vi "Ex-2 RT.vi"() -> ()   [LabVIEW 2014]
uses:
  <vilib>/NI/cRIO Wfm/ChannelConfig.ctl
  <vilib>/FPGAPlugInAG/sbRIO-9651/niLvFpga_Open_sbRIO-9651.vi
  <vilib>/rvi/interface/common/dynamic/niFpgaDynamicAddResources.vi
  <vilib>/FPGAPlugInAG/Dynamic/niLvFpga_Reset_Dynamic.vi
  <vilib>/FPGAPlugInAG/Dynamic/niLvFpga_Run_Dynamic.vi
  <vilib>/Utility/error.llb/Error Cluster From Error Code.vi
  <vilib>/rvi/errors/niLvFpgaAdjustHostInterfaceError.vi
  <vilib>/NI/cRIO Wfm/AcqRead(Wfm).vi
  <vilib>/FPGAPlugInAG/Dynamic/niLvFpga_Close_Dynamic.vi
  <vilib>/rvi/interface/nirviOpenFPGA/nirviOpenFPGA.xnode
  FPGA Bitfiles/SOMHands-ON_FPGATarget_Ex-2FPGASoln_+o7aZEmXAhs.lvbitx
  <vilib>/rvi/interface/nirviMethod/nirviMethod.xnode
  <vilib>/rvi/interface/nirviReadWriteControl/nirviReadWriteControl.xnode
  <vilib>/rvi/interface/nirviCloseFPGA/nirviCloseFPGA.xnode
  <vilib>/NI/cRIO Wfm/cRIO Wfm.lvlib
  NiFpgaLv.dll
  <vilib>/rvi/interface/Simulation/niFpgaSimulationCallBeginRW.vi
panel:
  in  "SPI PHY Settings":T1={"Divide Value"=10, "Transfer Length (bits)"=16, "CS Asserted Polarity"=FALSE, "Clock Polarity (CPOL)"=FALSE, "Clock Phase (CPHA)"=FALSE, "Lengthen MISO Setup"=FALSE, "Direction Change Bit"=0, "MOSI Starts as Output"=FALSE, "Tristatable MOSI"=FALSE}
  out "Acquired Data":waveform(sgl)[](graph)
  in  "scan rate [S/s]":u32=25000
  in  "quit":bool
  in  "number of samples":i32=2000 min=128
  in  "Samples per Channel":i32=1000
  # "Channel Settings"
  # "VI Controls"
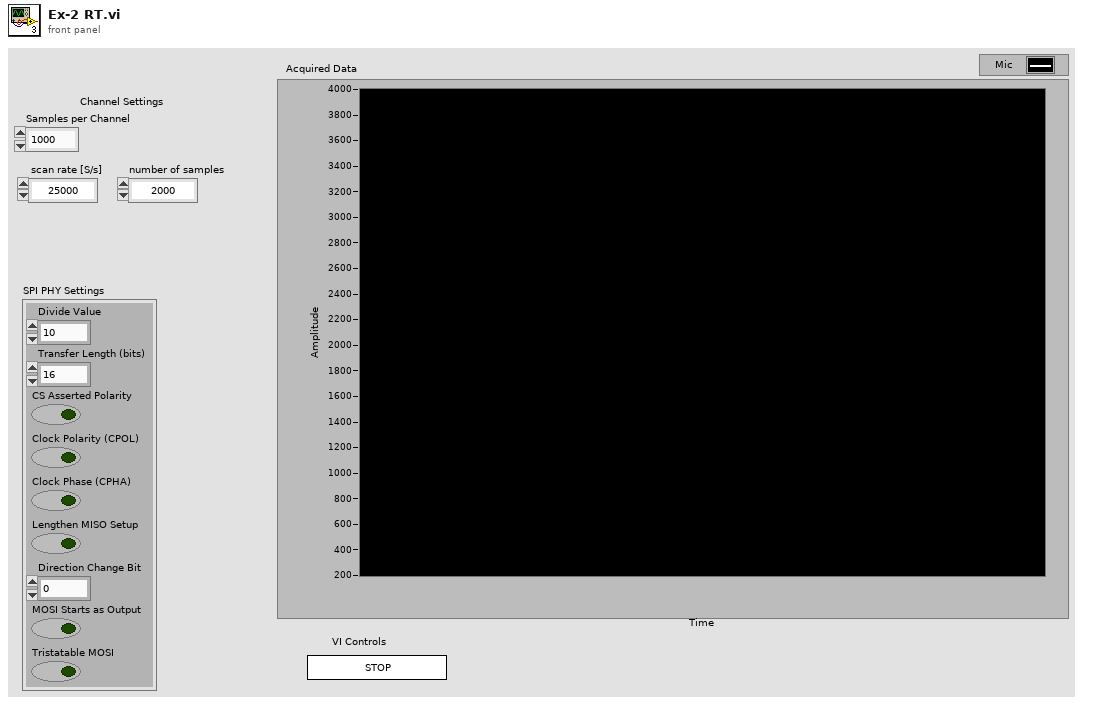
[diagram p1: front panel]
types:
  T1 = cluster{"Divide Value":u8, "Transfer Length (bits)":u8, "CS Asserted Polarity":bool, "Clock Polarity (CPOL)":bool, "Clock Phase (CPHA)":bool, "Lengthen MISO Setup":bool, "Direction Change Bit":u8, "MOSI Starts as Output":bool, "Tristatable MOSI":bool}
  T2 = typedef "cRIO Wfm.lvlib/ChannelConfig.ctl" = cluster{"Channel Name":string, "Sensitivity mV_EU":dbl, "EU":string, "dB Ref EU":dbl}[]
  T3 = typedef "cRIO Wfm.lvlib/SamplingInfo.ctl" = cluster{"Number of Channels":i32, "Actual Samp Rate":dbl, "Chan Name Array":string[], "EU Chan Array":string[], "dB Ref Chan Array":dbl[]}
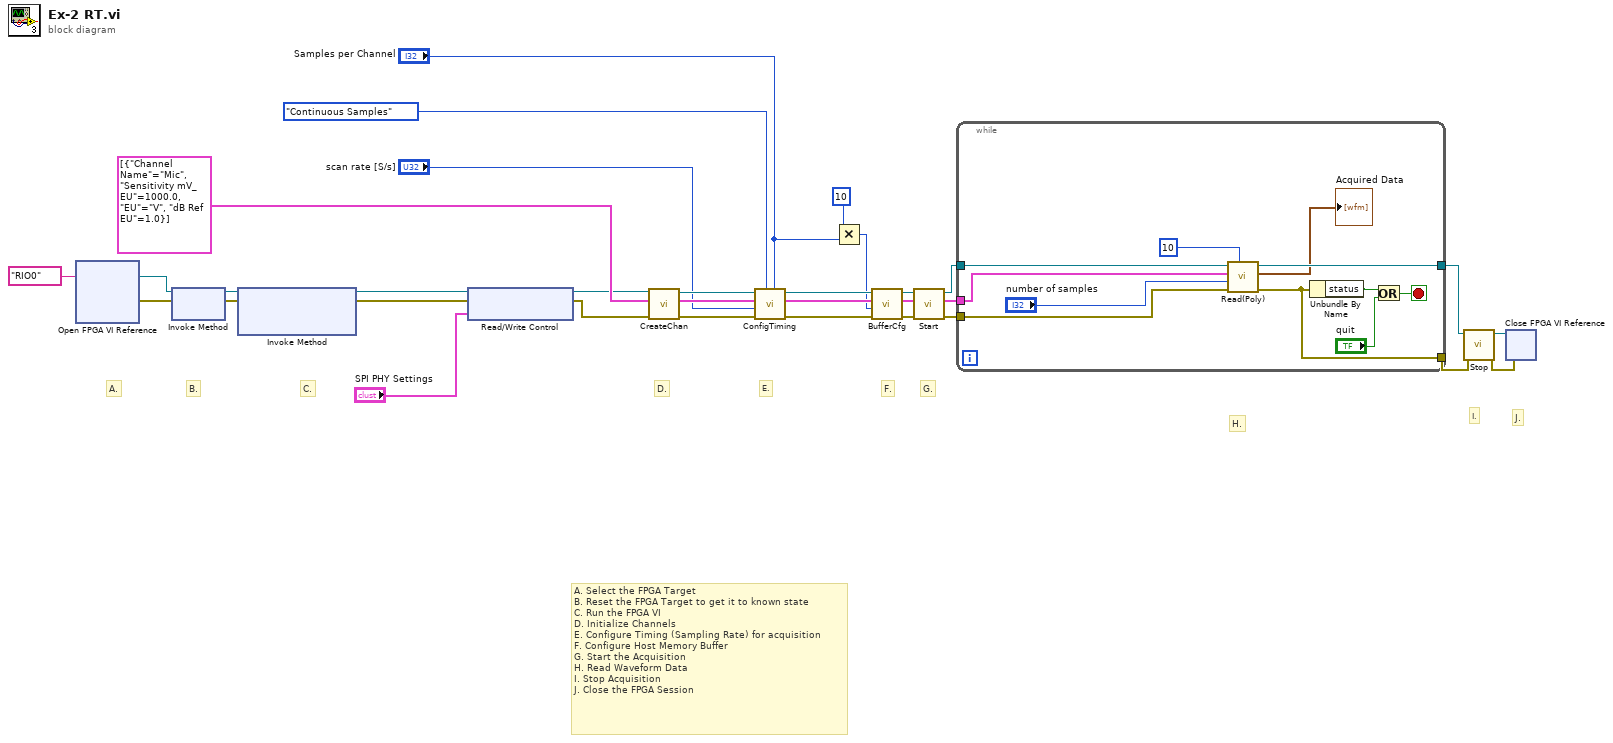
[diagram p0: block diagram]
diagram:
  # "A. Select the FPGA Target\nB. Reset the FPGA Target to get it to known state\nC. Run the FPGA VI\nD. Initialize Channels\nE. Configure Timing (Sampling Rate) for acquisition\nF. Configure Host Memory Buffer\nG. Start the Acquisition\nH. Read Waveform Data\nI. Stop Acquisition\nJ. Close the FPGA Session"
  # "J."
  # "I."
  # "H."
  # "G."
  # "F."
  # "E."
  # "D."
  # "C."
  # "B."
  # "A."
  n1 = xnode "Open FPGA VI Reference"("resource name"=tag "RIO0") -> ("FPGA VI Reference Out"=w18:refnum<k20>, "error out"=w19:errorcluster)  [unwired: 1 in]
  n2 = xnode "Invoke Method"("FPGA VI Reference In"=w18, "error in"=w19) -> ("FPGA VI Reference Out"=w17:refnum<k20>, "error out"=w16:errorcluster)
  n3 = xnode "Invoke Method"("FPGA VI Reference In"=w17, "error in"=w16) -> ("FPGA VI Reference Out"=w5:refnum<k20>, "error out"=w3:errorcluster)  [unwired: 1 in]
  n4 = xnode "Read/Write Control"("FPGA VI Reference In"=w5, "error in"=w3, "SPI PHY Settings"="SPI PHY Settings") -> ("FPGA VI Reference Out"=w4:refnum<k20>, "error out"=w2:errorcluster)
  n5 = call <vilib>:"CreateChan.vi"("error in"=w2, "Channel Info"=T2 [{"Channel Name"="Mic", "Sensitivity mV_EU"=1000.0, "EU"="V", "dB Ref EU"=1.0}], "Dynamic FPGA Ref"=w4) -> ("error out"=w22:errorcluster, "Sampling Info"=w26:T3, "Dynamic FPGA Ref Out"=w32:refnum<k20>)  [unwired: 6 in]
  n6 = call <vilib>:"ConfigTiming.vi"("Samples per Channel"="Samples per Channel", "Sample Mode"=enum16{"Finite Samples", "Continuous Samples"}."Continuous Samples", "error in"=w22, "Sample Rate"="scan rate [S/s]", "Sampling Info In"=w26, "Dynamic FPGA Ref"=w32) -> ("error out"=w21:errorcluster, "Sampling Info Out"=w27:T3, "Dynamic FPGA Ref Out"=w31:refnum<k20>)  [unwired: 2 in, 1 out]
  n7 = Multiply(x=10, y="Samples per Channel") -> (x*y=w23:i32)
  n8 = call <vilib>:"BufferCfg.vi"("error in"=w21, "Buffer Size [Samps per Chan]"=w23, "Sampling Info In"=w27, "Dynamic FPGA Ref"=w31) -> ("error out"=w20:errorcluster, "Sampling Info Out"=w25:T3, "Dynamic FPGA Ref Out"=w30:refnum<k20>)  [unwired: 4 in, 1 out]
  n9 = call <vilib>:"Start.vi"("error in"=w20, "Sampling Info In"=w25, "Dynamic FPGA Ref"=w30) -> ("error out"=w8:errorcluster, "Sampling Info Out"=w7:T3, "Dynamic FPGA Ref Out"=w9:refnum<k20>)  [unwired: 6 in]
  n10 = while {
    tunnel: [w35] -> w11
    tunnel: [w40] -> w12
    tunnel: w9 -> [w33]
    tunnel: w8 -> [w38]
    tunnel: w7 -> [w36]
    stop <- w42 stop-if-true
    n11 = call-poly <vilib>:"Read(Poly).vi"("Poll Time (ms)"=u32 10, "error in"=w38, "Samps Read per Chan"="number of samples", "Sampling Info"=w36, "Dynamic FPGA Ref"=w33) -> ("error out"=w35:errorcluster, "Wfm Data"=→"Acquired Data":waveform(sgl)[], "Dynamic FPGA Ref Out"=w40:refnum<k20>)  [unwired: 3 in, 1 out]
    n12 = Unbundle By Name(w35) -> ("status"=w41:bool)
    n13 = Or(x=w41, y="quit") -> (x .or. y?=w42:bool)
  }
  n14 = call <vilib>:"Stop.vi"("error in"=w11, "Dynamic FPGA Ref"=w12) -> ("error out"=w14:errorcluster, "Dynamic FPGA Ref Out"=w15:refnum<k20>)  [unwired: 8 in]
  n15 = xnode "Close FPGA VI Reference"("FPGA VI Reference In"=w15, "error in"=w14) -> ()  [unwired: 1 out]
